vi "Actor Core.vi"(8 "error in":errorcluster, 11 "Nested in":refnum<class "Interactor.lvclass">) -> (0 "error out":errorcluster, 3 "Actor out":refnum<class "Actor.lvclass">)   [LabVIEW 2024, in "Interactor.lvlib" / "Interactor.lvclass"]
doc: "(<B>Filename</B>: Actor Framework.lvlib:Actor.lvclass:Actor Core.vi)\n\nReceives messages to the actor, reacts to them, and initiates any error handling that may shut the actor down.\n\nDescendant classes may override this VI to append parallel tasks for the actor to complete while it handles messages. Overrides use the Call Parent Method node."
uses:
  Interactor.lvclass
  Interactor.lvclass/Interactor.ctl
  <vilib>/ActorFramework/Stop Msg/Stop Msg.lvclass
  <vilib>/MGI/Panel Manager/Panel Actor/Panel Actor/Panel Actor.lvclass
  Example/Home/Home.lvclass
  <vilib>/MGI/Panel Manager/Panel/Panel.lvlib
  <vilib>/MGI/Panel Manager/Panel/Panel/Subpanel/Subpanel.vi
  <vilib>/MGI/Panel Manager/Panel/Panel/Subpanel/Subpanel.lvclass
  Interactor Messages/Show Nested Panel Msg/Show Nested Panel Msg.lvclass
  Object Dictionary/Object Dictionary.lvclass
  HAL/HAL/Protocols/ICAN/ICAN.lvclass
  <vilib>/ActorFramework/Actor/Actor.lvclass
panel:
  in  "Copy Log Button":bool
  out "Log":string
  in  "Object Dictionary":bool
  in  "Home Button":bool
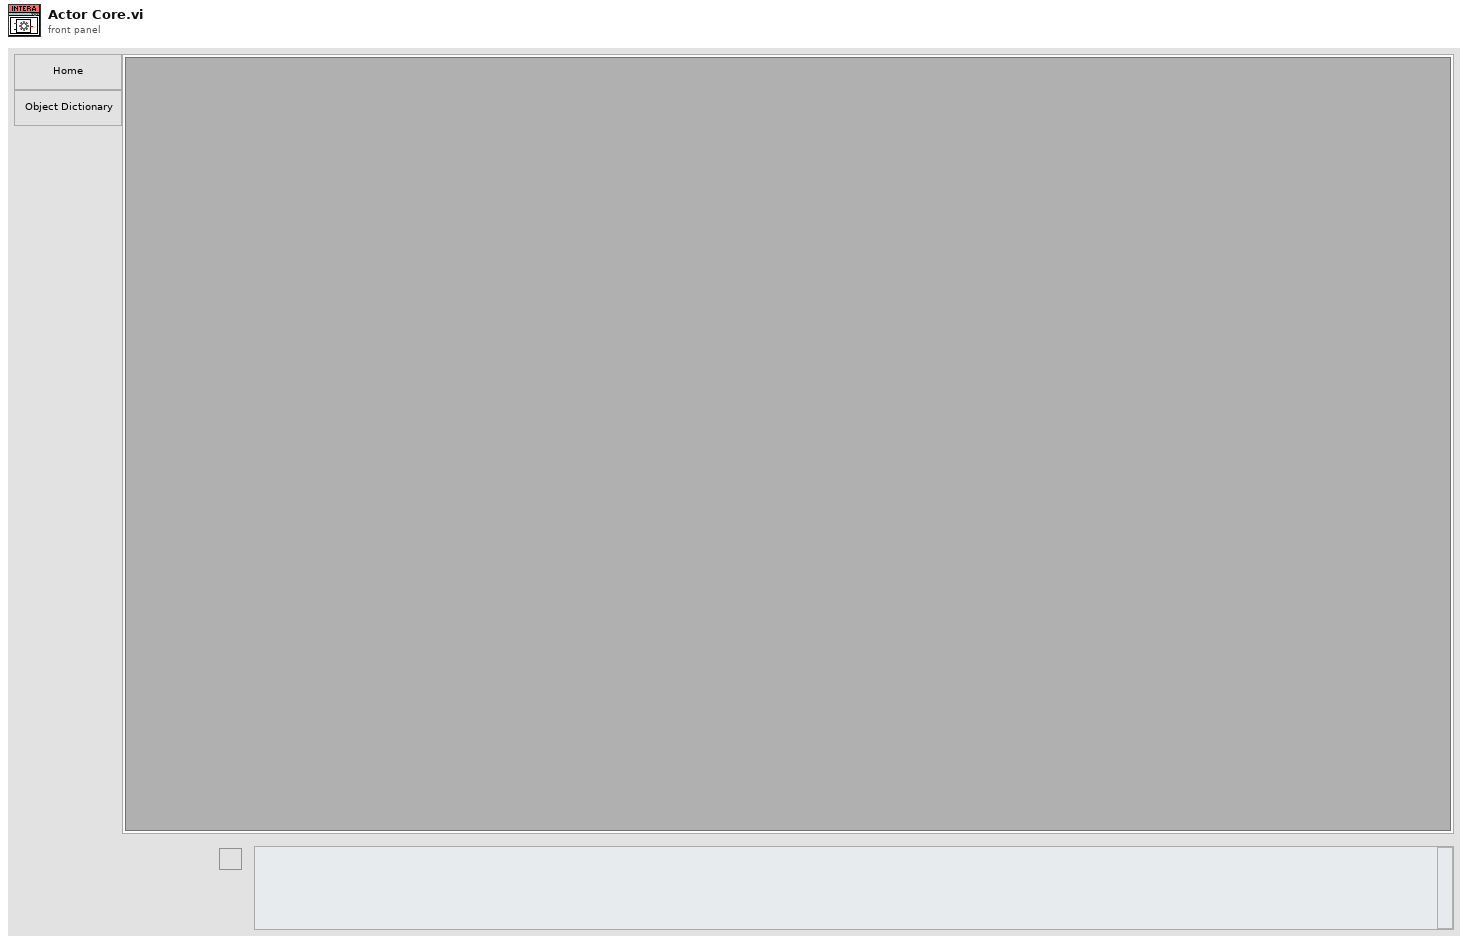
[diagram p1: front panel]
types:
  T1 = cluster{"Pnl Actor":refnum<event-registration>, "Event Registration Refnum":refnum<event-registration>}
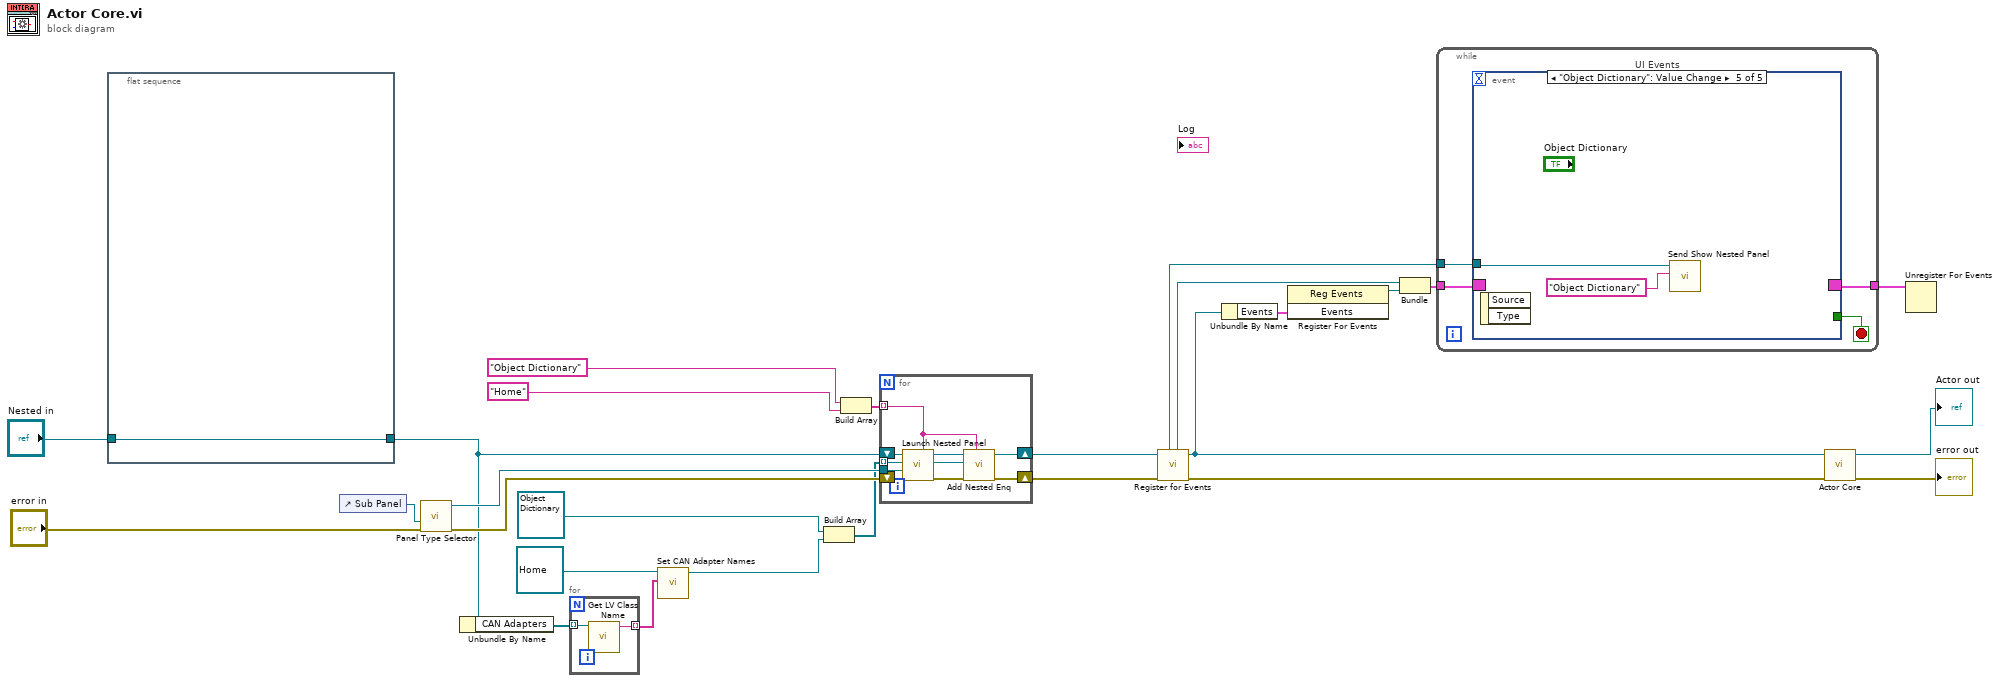
[diagram p0: block diagram]
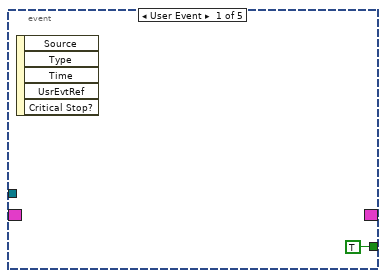
[diagram p2: hidden frame]
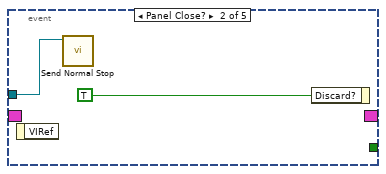
[diagram p3: hidden frame]
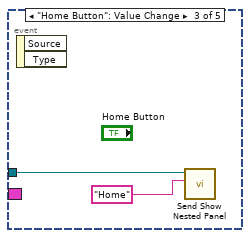
[diagram p4: hidden frame]
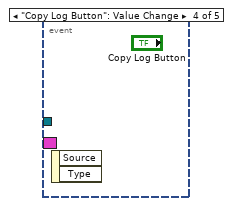
[diagram p5: hidden frame]
diagram:
  n1 = flat-sequence {
    tunnel: "Nested in" -> [w28]
    tunnel: [w28] -> w5
    frame #0 {
    }
  }
  n2 = control-ref of="Sub Panel"() -> (w17:refnum<vi>)
  n3 = call-poly <vilib>:"Panel Type Selector.vi"("Error In"="error in", "Sub Panel"=w17) -> ("Error Out"=w15:errorcluster, "Subpanel Out"=w11:refnum<class "Subpanel.lvclass">)  [unwired: 8 in]
  n4 = Unbundle By Name(w5) -> ("CAN Adapters"=w4:refnum<class "ICAN.lvclass">[])
  n5 = for {
    tunnel: w4 -> [w30] mode=indexing
    tunnel: [w29] -> w1 mode=indexing
    n6 = call <vilib>:"Get LV Class Name.vi"("object"=w30) -> ("class name"=w29:string)  [unwired: 9 in, 1 out]
  }
  n7 = call "Set CAN Adapter Names.vi"("CAN Adapter Names"=w1, "Home in"=refnum<class "Home.lvclass"> refnum ("Home.lvlib:Home.lvclass")) -> ("Home out"=w2:refnum<class "Home.lvclass">)  [unwired: 9 in]
  n8 = Build Array(refnum<class "Object Dictionary.lvclass"> refnum ("Object Dictionary.lvlib:Object Dictionary.lvclass"), w2) -> (w10:refnum<class "Panel Actor.lvclass">[])
  n9 = Build Array("Object Dictionary" ("Debug Alias"), "Home" ("Debug Alias")) -> (w9:string[])
  n10 = for {
    tunnel: w11 -> [w33]
    shift-right: [w37] -> w14
    shift-left: w15 -> [w39]
    shift-right: [w34] -> w12
    shift-left: w5 -> [w38]
    tunnel: w10 -> [w32] mode=indexing
    tunnel: w9 -> [w31] mode=indexing
    n11 = call <vilib>:"Launch Nested Panel.vi"("Debug Alias"=w31, "error in (no error)"=w39, "Panel"=w33, "Nested Panel Actor"=w32, "Panel Actor in"=w38) -> ("error out"=w37:errorcluster, "Nested Actor's Enqueuer"=w35:refnum<class "Message Enqueuer.lvclass">, "Panel Actor out"=w36:refnum<class "Interactor.lvclass">)  [unwired: 3 in, 1 out]
    n12 = call "Add Nested Enq.vi"("Ident"=w31, "Nested Actor's Enqueuer"=w35, "Interactor in"=w36) -> ("Interactor out"=w34:refnum<class "Interactor.lvclass">)  [unwired: 8 in]
  }
  n13 = call <vilib>:"Register for Events.vi"("Error In"=w14, "Panel Actor in"=w12) -> ("Error Out"=w19:errorcluster, "Panel Actor out"=w13:refnum<class "Interactor.lvclass">, "Pnl Actor"=w20:refnum<event-registration>, "Self Enqueuer"=w23:refnum<class "Message Enqueuer.lvclass">)  [unwired: 6 in]
  n14 = Unbundle By Name(w13) -> ("Events"=w25:cluster{"Stop":refnum<user-event>})
  n15 = register-events ("Main Register for Events")(w25) -> (reference out=w21:refnum<event-registration>)  [unwired: 2 in, 1 out]
  n16 = Bundle("Pnl Actor"=w20, "Event Registration Refnum"=w21) -> (w22:T1)  [unwired: 1 in]
  n17 = while {
    tunnel: w22 -> [w43]
    tunnel: [w41] -> w24
    tunnel: w23 -> [w40]
    stop <- w42 stop-if-true
    n18 = event "UI Events" shown="[4] \"Object Dictionary\": Value Change" {
      selector: w43 -> [_ _ _ _ _]
      dyn-events: [_ _ _ _ _] -> w41
      timeout: _ -> [_ _ _ _ _]
      tunnel: [TRUE _ _ _ _] -> w42
      tunnel: w40 -> [_ w45 w48 _ w49]
      event User Event {
        n19 = event-data() -> ()  [unwired: 1 in, 5 out]
      }
      event Panel Close? {
        n20 = event-data() -> ()  [unwired: 1 in, 1 out]
        n21 = call <vilib>:"Send Normal Stop.vi"("Message Enqueuer"=w45) -> ()  [unwired: 10 in, 1 out]
        n22 = event-data("Discard?"=TRUE) -> ()  [unwired: 1 in, 1 out]
      }
      event "Home Button": Value Change {
        n23 = event-data() -> ()  [unwired: 1 in, 2 out]
        n24 = call "Send Show Nested Panel.vi"("Ident"="Home", "Message Enqueuer"=w48) -> ()  [unwired: 8 in, 2 out]
      }
      event "Copy Log Button": Value Change {
        n25 = event-data() -> ()  [unwired: 1 in, 2 out]
      }
      event "Object Dictionary": Value Change {
        n26 = event-data() -> ()  [unwired: 1 in, 2 out]
        n27 = call "Send Show Nested Panel.vi"("Ident"="Object Dictionary", "Message Enqueuer"=w49) -> ()  [unwired: 8 in, 2 out]
      }
    }
  }
  n28 = call-parent "Actor Core.vi"("error in"=w19, "Panel Actor in"=w13) -> ("error out"=→"error out":errorcluster, "Actor out"=→"Actor out":refnum<class "Actor.lvclass">)  [unwired: 8 in]
  n29 = Unregister For Events(event registration refnum=w24) -> ()  [unwired: 1 in, 1 out]
